vi "Get Tx Scheduled Label Configuration.vi"(8 "error in":errorcluster, 10 "configuration string":string, 11 "port":T1 format="%.0x") -> (0 "error out":errorcluster, 2 "configuration string out":string, 3 "port out":T1 format="%.0x")   [LabVIEW 2020, in "Ballard ARINC 429 Hardware Configuration.lvlib"]
uses:
  Ballard ARINC 429 Hardware Configuration.lvlib
  <vilib>/NI VeriStand/Custom Device API/Custom Device Item Ref.ctl
  Scripting/Ballard/Ballard ARINC 429 Scripting.lvlib
  Scripting/ARINC 429/ARINC 429 Scripting.lvlib
  <vilib>/NI VeriStand/Custom Device API/Custom Device API.lvlib
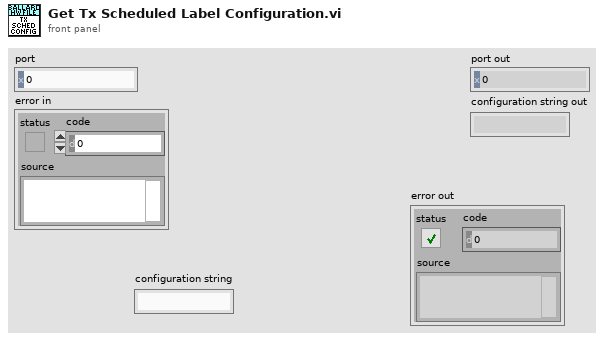
[diagram p1: front panel]
types:
  T1 = typedef "Custom Device API.lvlib/Custom Device Item Ref.ctl" = u64
  T2 = typedef "Label Properties.ctl" = cluster{"label (Dec)":T3, "SDI value":u8, "SDI enabled":bool}
  T3 = typedef "Label.ctl" = u8
  T4 = typedef "Transfer Type.ctl" = enum16{"Scheduled", "Acyclic", "Block", "Strobe"}
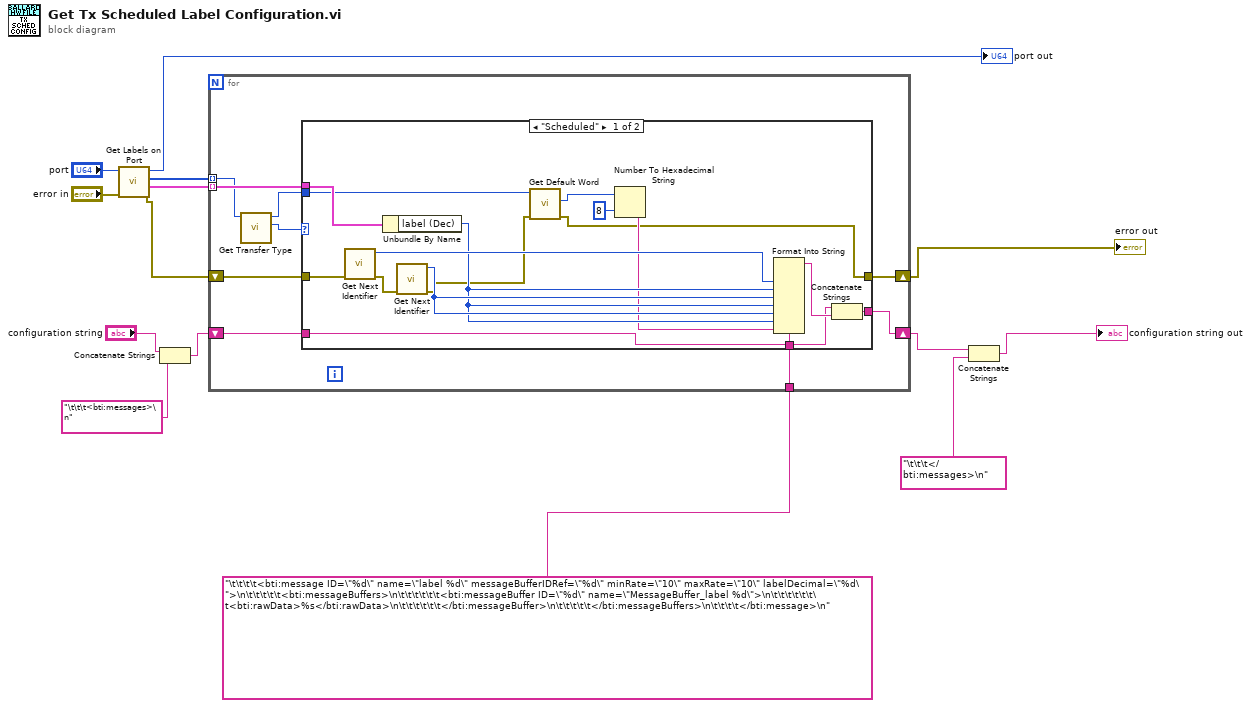
[diagram p0: block diagram]
diagram:
  n1 = call "Get Labels on Port.vi"("error in"="error in", "port in"="port") -> ("error out"=w5:errorcluster, "labels properties"=w8:T2[], "labels"=w7:T1[], "port out"=→"port out":T1)  [unwired: 6 in]
  n2 = Concatenate Strings("configuration string", "\t\t\t<bti:messages>\n") -> (w9:string)
  n3 = for {
    shift-right: [w19] -> w3
    shift-left: w9 -> [w20]
    tunnel: w8 -> [w22] mode=indexing
    tunnel: w7 -> [w17] mode=indexing
    tunnel: "\t\t\t\t<bti:message ID=\"%d\" name=\"label %d\" messageBufferIDRef=\"%d\" minRate=\"10\" maxRate=\"10\" labelDecimal=\"%d\">\n\t\t\t\t\t<bti:messageBuffers>\n\t\t\t\t\t\t<bti:messageBuffer ID=\"%d\" name=\"MessageBuffer_label %d\">\n\t\t\t\t\t\t\t<bti:rawData>%s</bti:rawData>\n\t\t\t\t\t\t</bti:messageBuffer>\n\t\t\t\t\t</bti:messageBuffers>\n\t\t\t\t</bti:message>\n" -> [w23]
    shift-right: [w18] -> w4
    shift-left: w5 -> [w21]
    n4 = call "Get Transfer Type.vi"("label ref in"=w17) -> ("transfer type"=w15:T4, "label ref out"=w16:T1)  [unwired: 8 in, 1 out]
    n5 = case shown="\"Scheduled\"" w15 {
      tunnel: w23 -> [w39 _]
      tunnel: w22 -> [w38 _]
      tunnel: w21 -> [w37 w41]
      tunnel: w20 -> [w27 w40]
      tunnel: [w26 w40] -> w19
      tunnel: [w25 w41] -> w18
      tunnel: w16 -> [w24 _]
      frame "Scheduled" {
        n6 = call "Get Next Identifier.vi"("error in"=w37) -> ("error out"=w35:errorcluster, "ID"=w36:u32)  [unwired: 9 in]
        n7 = Unbundle By Name(w38) -> ("label (Dec)"=w33:T3)
        n8 = call "Get Next Identifier.vi"("error in"=w35) -> ("error out"=w32:errorcluster, "ID"=w34:u32)  [unwired: 9 in]
        n9 = call "Get Default Word.vi"("error in"=w32, "Item Ref in"=w24) -> ("error out"=w25:errorcluster, "default word"=w31:u32)  [unwired: 7 in, 1 out]
        n10 = Number To Hexadecimal String(1:i16 8 ("width (-)"), 2:w31) -> (0:w29:string)
        n11 = Format Into String(format string=w39, w36, w33, w34, w33, w34, w33, w29) -> (resulting string=w28:string)  [unwired: 2 in, 1 out]
        n12 = Concatenate Strings(w27, w28) -> (w26:string)
      }
      frame Default {
      }
    }
  }
  "error out" <- w4
  n13 = Concatenate Strings(w3, "\t\t\t</bti:messages>\n") -> (→"configuration string out":string)
